vi "Update V.vi"(8 "error in (no error)":errorcluster, 10 "SLAM In":T3, 11 "New LM's In":T2(array[cluster])) -> (0 "error out":errorcluster, 2 "SLAM Out":T3, 3 "New LM's Out":T2(array[cluster]))   [LabVIEW 2009]
uses:
  <vilib>/Analysis/Matrix/Datatypes/RealMatrix.ctl
  Controls/SLAM.ctl
  <vilib>/Analysis/Matrix/NI_Matrix.lvlib
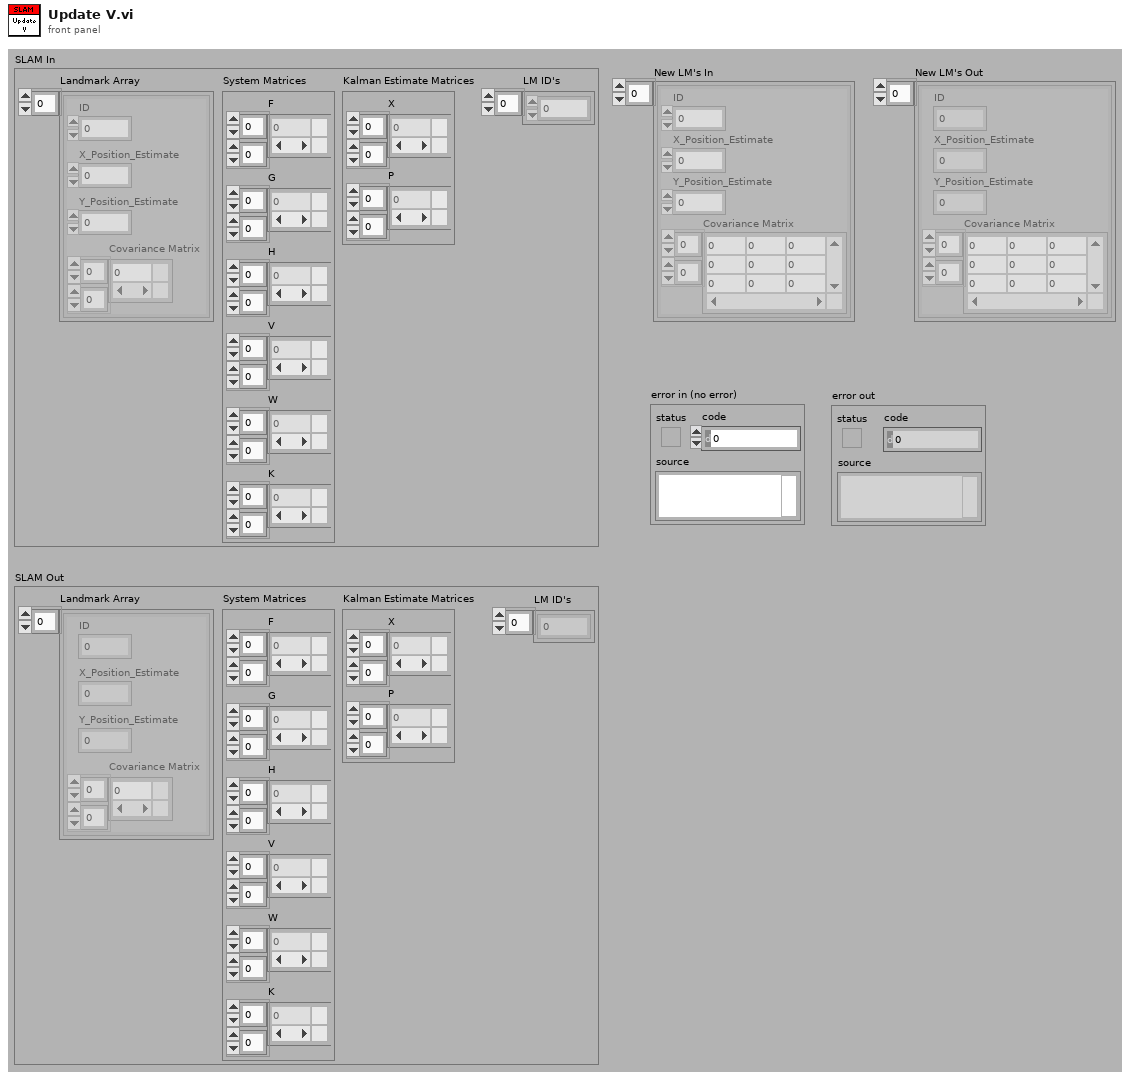
[diagram p1: front panel]
types:
  T1 = typedef "NI_Matrix.lvlib/RealMatrix.ctl" = dbl[][]
  T2 = cluster{"ID":dbl, "X_Position_Estimate":dbl, "Y_Position_Estimate":dbl, "Covariance Matrix":T1}[]
  T3 = typedef "SLAM.ctl" = cluster{"Landmark Array":cluster{"ID":dbl, "X_Position_Estimate":dbl, "Y_Position_Estimate":dbl, "Covariance Matrix":T1}[], "System Matrices":cluster{"F":T1, "G":T1, "H":T1, "V":T1, "W":T1, "K":T1}, "Kalman Estimate Matrices":cluster{"X":T1, "P":T1}, "LM ID's":dbl[]}
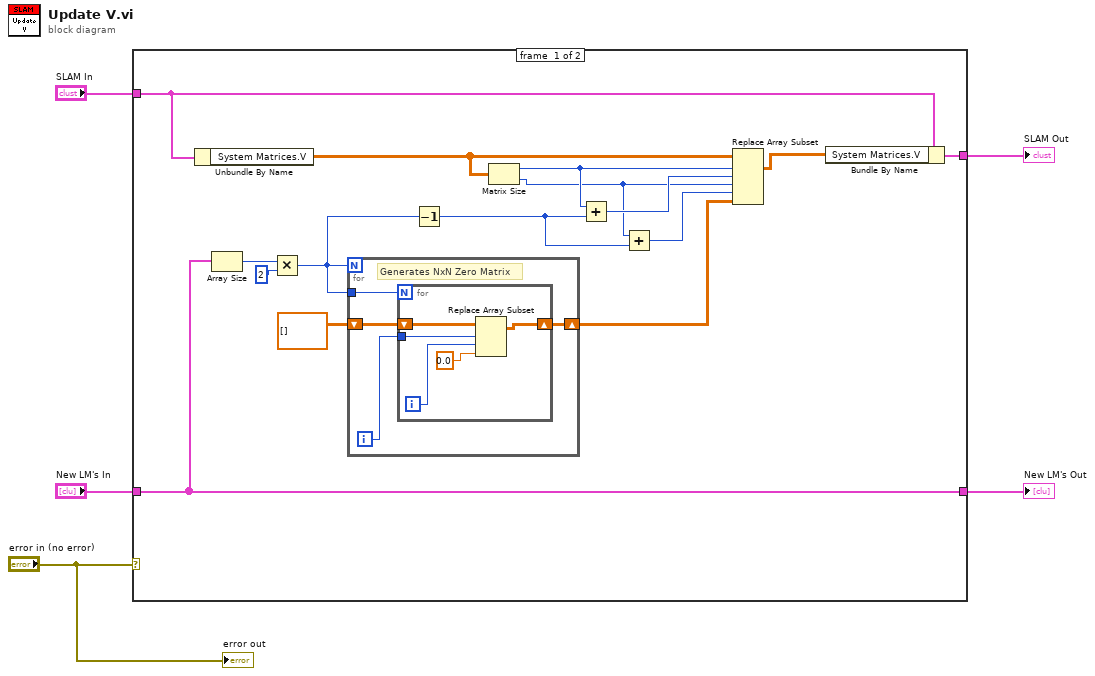
[diagram p0: block diagram]
diagram:
  n1 = case shown="No Error" "error in (no error)" {
    tunnel: "SLAM In" -> [w19 w30]
    tunnel: "New LM's In" -> [w9 w31]
    tunnel: [w12 w30] -> w3
    tunnel: [w9 w31] -> w2
    frame #0 {
      n2 = Unbundle By Name(w19) -> ("System Matrices.V"=w10:T1)
      n3 = Array Size(array=w9) -> (size(s)=w8:i32)
      n4 = Multiply(x=w8, y=2) -> (x*y=w7:i32)
      n5 = for {
        N: w7 -> [_]
        tunnel: w7 -> [w24]
        shift-right: [w21] -> w14
        shift-left: T1 [] ("matrix") -> [w23]
        i -> [w22]
        # "Generates NxN Zero Matrix"
        n6 = for {
          N: w24 -> [_]
          shift-right: [w28] -> w21
          shift-left: w23 -> [w29]
          tunnel: w22 -> [w27]
          i -> [w26]
          n7 = Replace Array Subset(array=w29, new element=0.0 ("new element/submatrix"), index (row)=w27, index (col)=w26) -> (w28:T1)
        }
      }
      n8 = Decrement(x=w7) -> (x-1=w13:i32)
      n9 = Matrix Size(0:w10) -> (1:w18:i32, 2:w16:i32)
      n10 = Add(x=w18, y=w13) -> (x+y=w17:i32)
      n11 = Add(x=w16, y=w13) -> (x+y=w15:i32)
      n12 = Replace Array Subset(array=w10, new element=w14, index (dim 0)=w18, index (dim 1)=w17, index (dim 2)=w16, index (dim 3)=w15) -> (w11:T1)
      n13 = Bundle By Name(cluster=w19, "System Matrices.V"=w11) -> (w12:T3)
    }
    frame #1 {
    }
  }
  "New LM's Out" <- w2
  "SLAM Out" <- w3
  "error out" <- "error in (no error)"
